vi "BEElab.vi"() -> ()   [LabVIEW 2010]
panel:
  in  "T 1":bool
  in  "T2":bool
  in  "T3":bool
  in  "T4":bool
  out "spreadsheet string":string
  in  "index 5":i32=83
  in  "index 4":i32=56
  out "error out":errorcluster
  in  "index":i32=18
  in  "index 2":i32=25
  in  "index 3":i32=52
  out "String 2":string
  out "Numeric":dbl
  out "in":i32
  out "String":string
  in  "Tab Control":enum32{"Load Profile", "View Data"}(tab)
  in  "Massachusetts - Winter":bool
  in  "Arizona  - Winter":bool
  in  "Massachusetts - Summer":bool
  in  "Arizona - Summer":bool
  out "Waveform Graph":dbl[](graph)
  in  "Weekend computer only":bool
  in  "0":dbl min=0.0 max=3.0 step=1.0
  in  "1":dbl min=0.0 max=3.0 step=1.0
  in  "2":dbl min=0.0 max=3.0 step=1.0
  in  "5":dbl min=0.0 max=3.0 step=1.0
  in  "4":dbl min=0.0 max=3.0 step=1.0
  in  "3":dbl min=0.0 max=3.0 step=1.0
  in  "11":dbl min=0.0 max=3.0 step=1.0
  in  "10":dbl min=0.0 max=3.0 step=1.0
  in  "9":dbl min=0.0 max=3.0 step=1.0
  in  "6":dbl min=0.0 max=3.0 step=1.0
  in  "7":dbl min=0.0 max=3.0 step=1.0
  in  "8":dbl min=0.0 max=3.0 step=1.0
  in  "15":dbl min=0.0 max=3.0 step=1.0
  in  "14":dbl min=0.0 max=3.0 step=1.0
  in  "13":dbl min=0.0 max=3.0 step=1.0
  in  "20":dbl min=0.0 max=3.0 step=1.0
  in  "19":dbl min=0.0 max=3.0 step=1.0
  in  "16":dbl min=0.0 max=3.0 step=1.0
  in  "17":dbl min=0.0 max=3.0 step=1.0
  in  "18":dbl min=0.0 max=3.0 step=1.0
  in  "23":dbl min=0.0 max=3.0 step=1.0
  in  "22":dbl min=0.0 max=3.0 step=1.0
  in  "21":dbl min=0.0 max=3.0 step=1.0
  in  "12":dbl min=0.0 max=3.0 step=1.0
  in  "Step Usage":bool
  in  "Office 9am - 5pm work day":bool
  in  "Launch Experiment":bool
  in  "Clear":bool
  out "Temperture":cluster{dbl, dbl, dbl, dbl}(graph)
  out "Usage Watts":cluster{dbl}(graph)
  in  "stop":bool
  out "Thermal Load Profile":dbl[](graph)
  # "Building Energy Efficiency iLab"
  # "Select the climate (currently externally controlled).\n\nUse the predefined configurations or custom configuration area\nto specify thermal load profiles for your experimnt.\n\nCLick the Save and Launch button to begin your experiment."
  # "Select a climate for the test chamber:"
  # "Predefined Configurations:"
  # "Custom Configurations:"
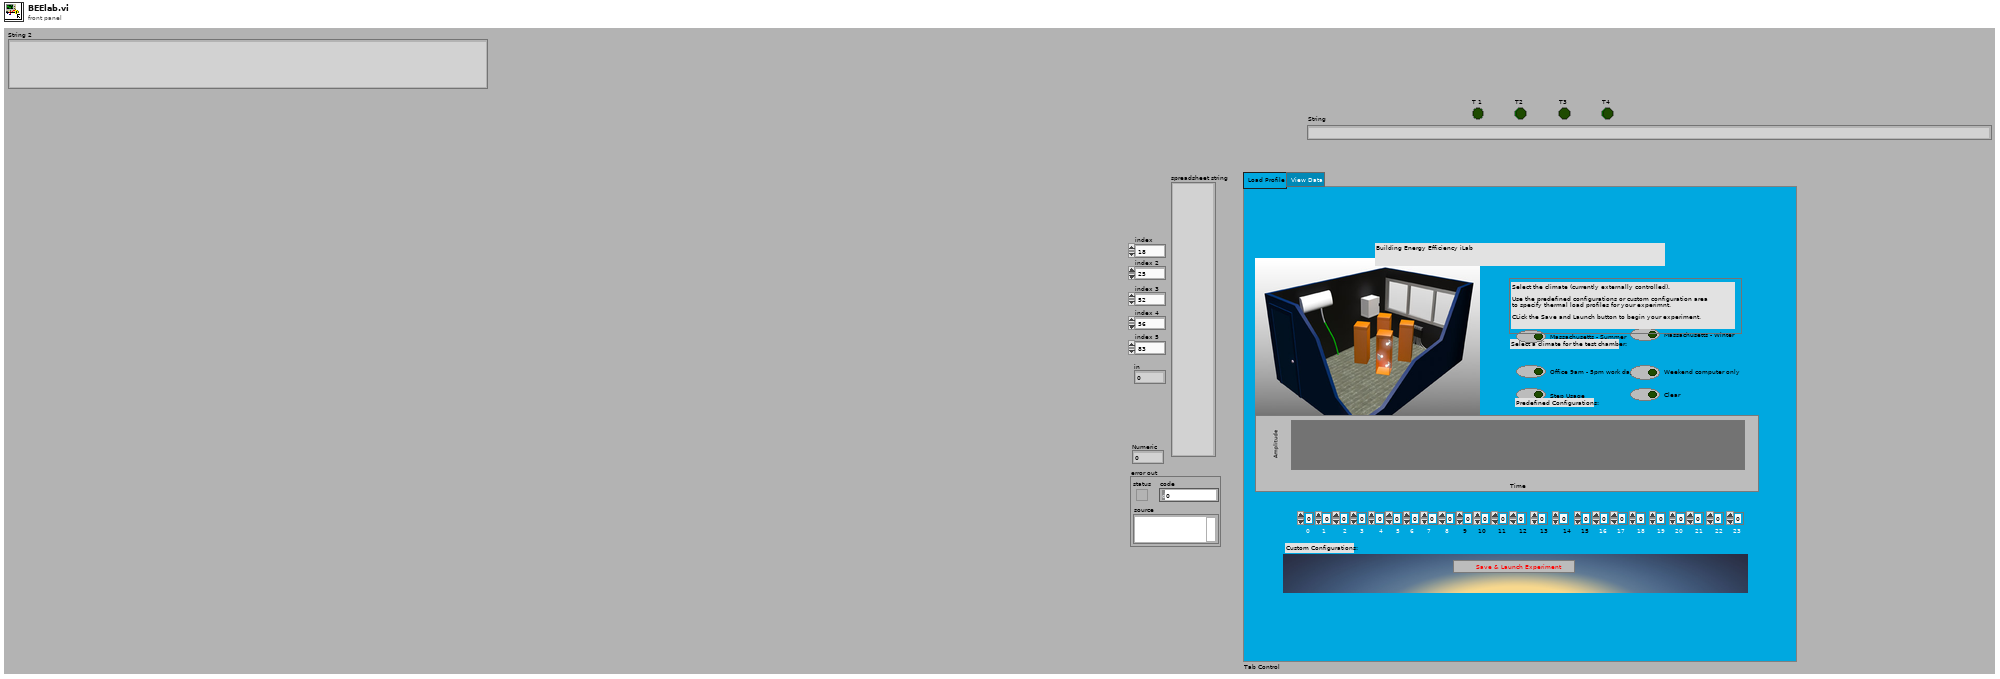
[diagram p1: front panel]
types:
  T1 = enum16{"Read", "Write", "ReadWrite", "BufferedRead", "BufferedReadWrite"}
  T2 = enum32{"Page Enabled", "Page Disabled", "Page Disabled & Grayed"}
  T3 = cluster{"0":dbl, "1":dbl, "2":dbl, "3":dbl, "4":dbl, "5":dbl, "6":dbl, "7":dbl, "8":dbl, "9":dbl, "10":dbl, "11":dbl, "12":dbl, "13":dbl, "14":dbl, "15":dbl, "16":dbl, "17":dbl, "18":dbl, "19":dbl, "20":dbl, "21":dbl, "22":dbl, "23":dbl}
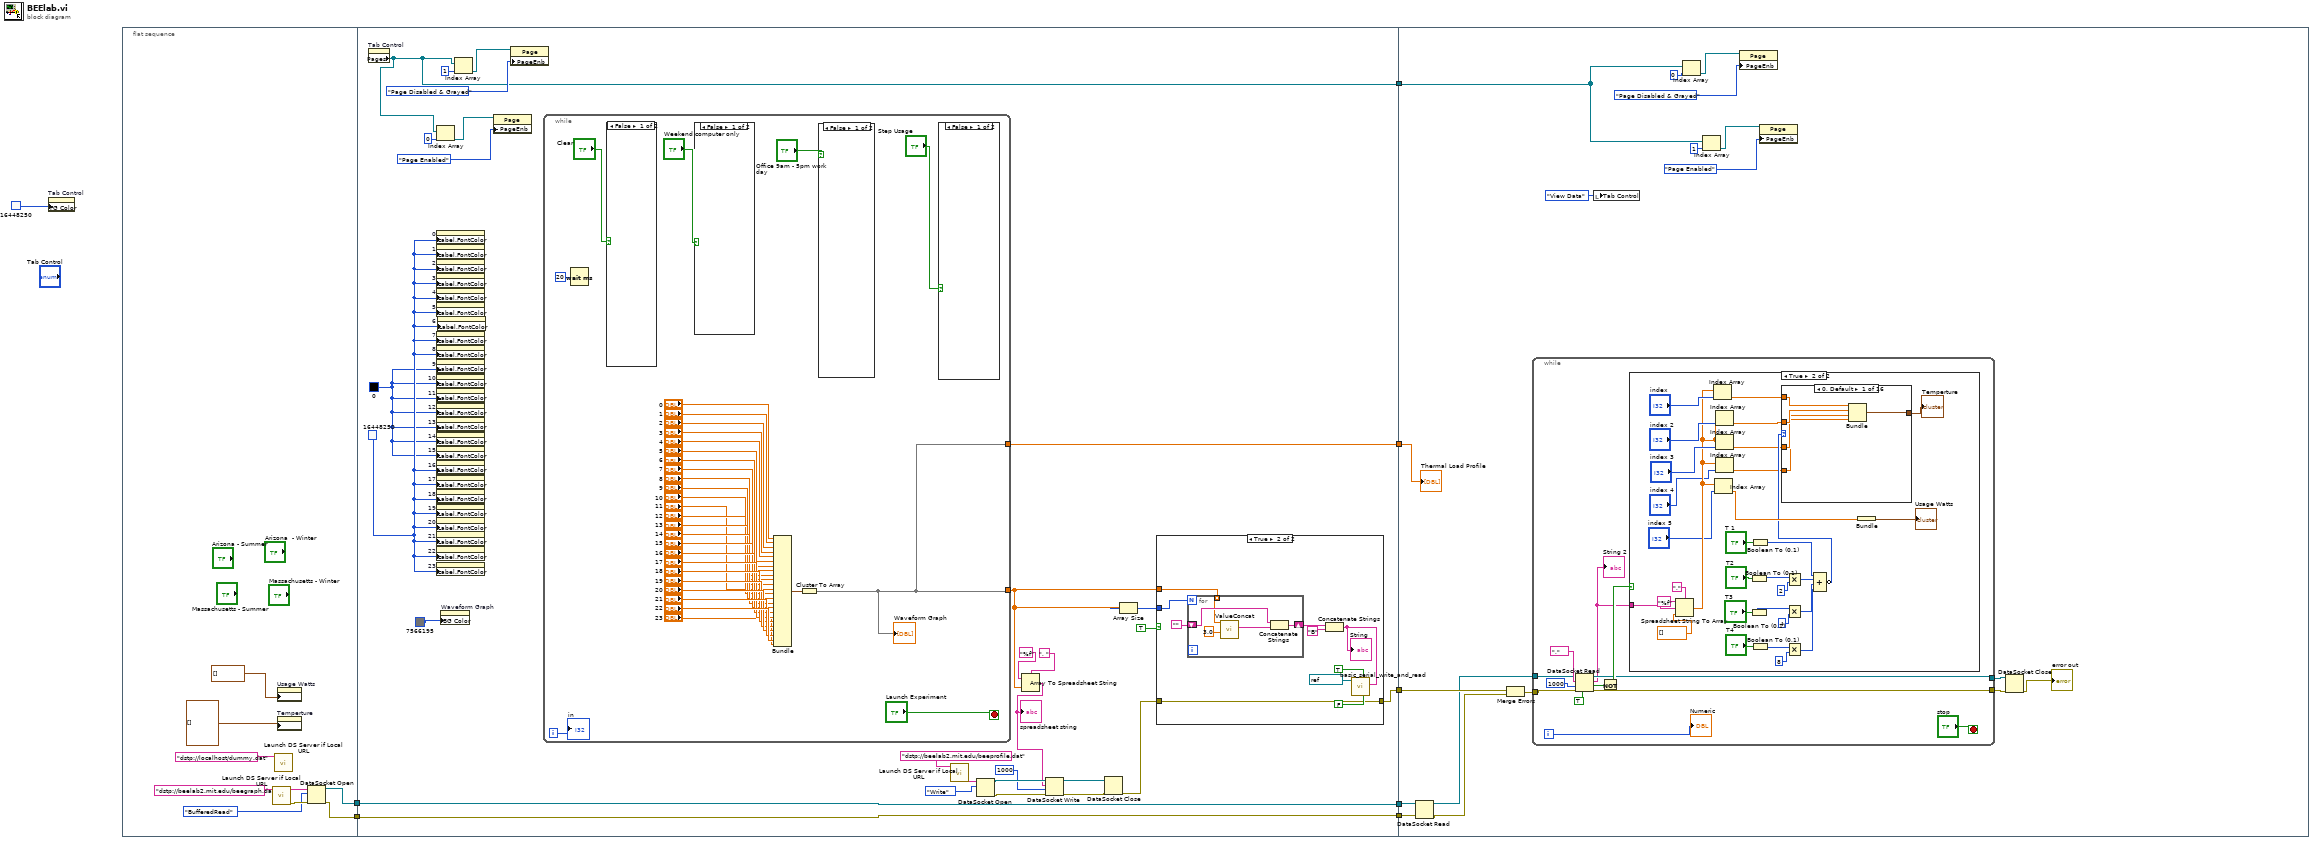
[diagram p0: block diagram]
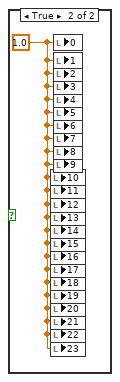
[diagram p3: hidden frame]
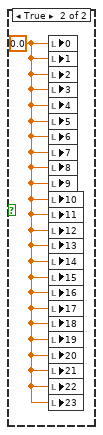
[diagram p4: hidden frame]
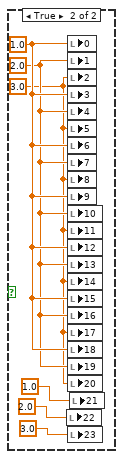
[diagram p5: hidden frame]
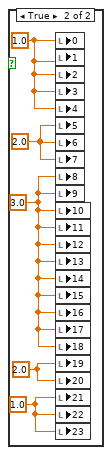
[diagram p6: hidden frame]
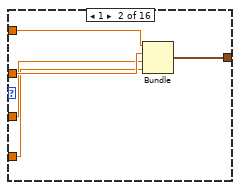
[diagram p8: hidden frame]
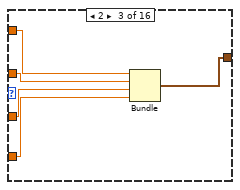
[diagram p9: hidden frame]
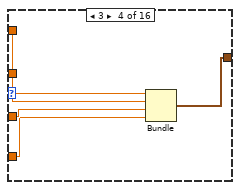
[diagram p10: hidden frame]
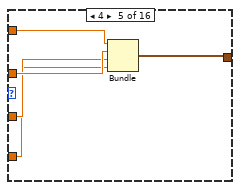
[diagram p11: hidden frame]
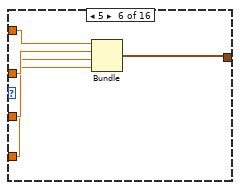
[diagram p12: hidden frame]
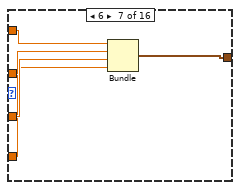
[diagram p13: hidden frame]
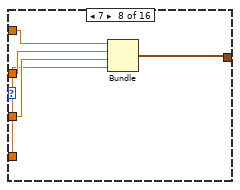
[diagram p14: hidden frame]
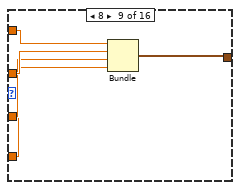
[diagram p15: hidden frame]
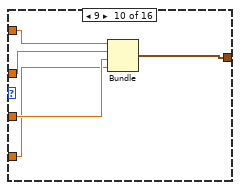
[diagram p16: hidden frame]
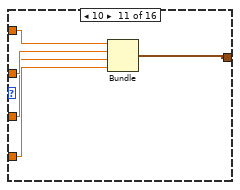
[diagram p17: hidden frame]
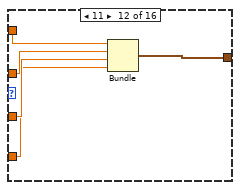
[diagram p18: hidden frame]
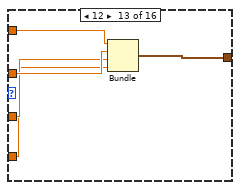
[diagram p19: hidden frame]
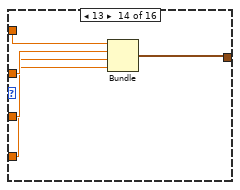
[diagram p20: hidden frame]
diagram:
  n1 = property on="Tab Control" class="TabCtl (strict)"("FG Color"=u32 16448250) -> ()  [unwired: 2 in, 2 out]
  n2 = flat-sequence {
    tunnel: [w12] -> w4
    tunnel: [w11] -> w2
    tunnel: [w36] -> w7
    tunnel: [w31] -> w6
    tunnel: [w30] -> w5
    tunnel: w4 -> [w29]
    tunnel: [w29] -> w3
    tunnel: w2 -> [w30]
    tunnel: [w18] -> w1
    tunnel: w7 -> [w122]
    tunnel: w6 -> [w115]
    tunnel: w5 -> [w110]
    tunnel: w3 -> [w109]
    tunnel: w1 -> [w114]
    frame #0 {
      n3 = call "Launch DS Server if Local URL.vi"("URL"="dstp://beelab2.mit.edu/beegraph.dat") -> ("error out"=w15:errorcluster, "Duplicate URL"=w16:string)  [unwired: 1 in, 4 out]
      n4 = call "Launch DS Server if Local URL.vi"("URL"="dstp://localhost/dummy.dat") -> ()  [unwired: 1 in, 6 out]
      n5 = property on="Usage Watts" class="WFChart (strict)"("History Data"=cluster{dbl}[] []) -> ()  [unwired: 2 in, 2 out]
      n6 = property on="Temperture" class="WFChart (strict)"("History Data"=cluster{dbl, dbl, dbl, dbl}[] []) -> ()  [unwired: 2 in, 2 out]
      n7 = DataSocket Open(8:w15, 10:T1."BufferedRead" ("mode"), 11:w16) -> (0:w12:errorcluster, 3:w11:refnum<k13>)  [unwired: 1 in]
    }
    frame #1 {
      w44 = u32 0
      w45 = u32 16448250
      n8 = property on="Tab Control" class="TabCtl (strict)"() -> ("Pages"=w36:refnum<vi>[])  [unwired: 2 in, 2 out]
      n9 = property on="15" class="DigNum (strict)"("Label.FontColor"=w44) -> ()  [unwired: 2 in, 2 out]
      n10 = property on="16" class="DigNum (strict)"("Label.FontColor"=w45) -> ()  [unwired: 2 in, 2 out]
      n11 = property on="17" class="DigNum (strict)"("Label.FontColor"=w45) -> ()  [unwired: 2 in, 2 out]
      n12 = property on="18" class="DigNum (strict)"("Label.FontColor"=w45) -> ()  [unwired: 2 in, 2 out]
      n13 = property on="19" class="DigNum (strict)"("Label.FontColor"=w45) -> ()  [unwired: 2 in, 2 out]
      n14 = property on="20" class="DigNum (strict)"("Label.FontColor"=w45) -> ()  [unwired: 2 in, 2 out]
      n15 = property on="21" class="DigNum (strict)"("Label.FontColor"=w45) -> ()  [unwired: 2 in, 2 out]
      n16 = Index Array(array=w36, index=0) -> (element=w42:refnum<vi>)
      n17 = property on="0" class="DigNum (strict)"("Label.FontColor"=w45) -> ()  [unwired: 2 in, 2 out]
      n18 = property on="1" class="DigNum (strict)"("Label.FontColor"=w45) -> ()  [unwired: 2 in, 2 out]
      n19 = property on="2" class="DigNum (strict)"("Label.FontColor"=w45) -> ()  [unwired: 2 in, 2 out]
      n20 = property on="3" class="DigNum (strict)"("Label.FontColor"=w45) -> ()  [unwired: 2 in, 2 out]
      n21 = property on="4" class="DigNum (strict)"("Label.FontColor"=w45) -> ()  [unwired: 2 in, 2 out]
      n22 = property on="5" class="DigNum (strict)"("Label.FontColor"=w45) -> ()  [unwired: 2 in, 2 out]
      n23 = property on="7" class="DigNum (strict)"("Label.FontColor"=w45) -> ()  [unwired: 2 in, 2 out]
      n24 = property on="8" class="DigNum (strict)"("Label.FontColor"=w45) -> ()  [unwired: 2 in, 2 out]
      n25 = property on="9" class="DigNum (strict)"("Label.FontColor"=w44) -> ()  [unwired: 2 in, 2 out]
      n26 = property on="10" class="DigNum (strict)"("Label.FontColor"=w44) -> ()  [unwired: 2 in, 2 out]
      n27 = property on="11" class="DigNum (strict)"("Label.FontColor"=w44) -> ()  [unwired: 2 in, 2 out]
      n28 = property on="12" class="DigNum (strict)"("Label.FontColor"=w44) -> ()  [unwired: 2 in, 2 out]
      n29 = property on="13" class="DigNum (strict)"("Label.FontColor"=w44) -> ()  [unwired: 2 in, 2 out]
      n30 = property on="14" class="DigNum (strict)"("Label.FontColor"=w44) -> ()  [unwired: 2 in, 2 out]
      n31 = property on="22" class="DigNum (strict)"("Label.FontColor"=w45) -> ()  [unwired: 2 in, 2 out]
      n32 = property on="23" class="DigNum (strict)"("Label.FontColor"=w45) -> ()  [unwired: 2 in, 2 out]
      n33 = property on="6" class="DigNum (strict)"("Label.FontColor"=w45) -> ()  [unwired: 2 in, 2 out]
      n34 = property on="Waveform Graph" class="WFGraph (strict)"("BG Color"=u32 7566195) -> ()  [unwired: 2 in, 2 out]
      n35 = Index Array(array=w36, index=1) -> (element=w41:refnum<vi>)
      n36 = property class="Page"(reference=w42, "PageEnb"=T2."Page Enabled" ("Page Enabled State")) -> ()  [unwired: 1 in, 2 out]
      n37 = property class="Page"(reference=w41, "PageEnb"=T2."Page Disabled & Grayed" ("Page Enabled State")) -> ()  [unwired: 1 in, 2 out]
      n38 = while {
        tunnel: [w63] -> w35
        tunnel: [w63] -> w18
        i -> [w66]
        stop <- "Launch Experiment" stop-if-true
        n39 = Wait (ms)(milliseconds to wait=u32 20) -> ()  [unwired: 1 out]
        n40 = case shown="False" "Clear" {
          frame False {
          }
          frame True {
            w97 = 0.0 ("0")
            n41 = local write "0"(w97) -> ()
            n42 = local write "1"(w97) -> ()
            n43 = local write "2"(w97) -> ()
            n44 = local write "3"(w97) -> ()
            n45 = local write "4"(w97) -> ()
            n46 = local write "5"(w97) -> ()
            n47 = local write "6"(w97) -> ()
            n48 = local write "7"(w97) -> ()
            n49 = local write "8"(w97) -> ()
            n50 = local write "9"(w97) -> ()
            n51 = local write "10"(w97) -> ()
            n52 = local write "11"(w97) -> ()
            n53 = local write "12"(w97) -> ()
            n54 = local write "13"(w97) -> ()
            n55 = local write "14"(w97) -> ()
            n56 = local write "15"(w97) -> ()
            n57 = local write "16"(w97) -> ()
            n58 = local write "17"(w97) -> ()
            n59 = local write "18"(w97) -> ()
            n60 = local write "19"(w97) -> ()
            n61 = local write "20"(w97) -> ()
            n62 = local write "21"(w97) -> ()
            n63 = local write "22"(w97) -> ()
            n64 = local write "23"(w97) -> ()
          }
        }
        n65 = case shown="False" "Weekend computer only" {
          frame False {
          }
          frame True {
            w96 = 1.0 ("0")
            n66 = local write "10"(w96) -> ()
            n67 = local write "11"(w96) -> ()
            n68 = local write "12"(w96) -> ()
            n69 = local write "13"(w96) -> ()
            n70 = local write "14"(w96) -> ()
            n71 = local write "15"(w96) -> ()
            n72 = local write "16"(w96) -> ()
            n73 = local write "17"(w96) -> ()
            n74 = local write "18"(w96) -> ()
            n75 = local write "19"(w96) -> ()
            n76 = local write "20"(w96) -> ()
            n77 = local write "21"(w96) -> ()
            n78 = local write "22"(w96) -> ()
            n79 = local write "23"(w96) -> ()
            n80 = local write "0"(w96) -> ()
            n81 = local write "1"(w96) -> ()
            n82 = local write "2"(w96) -> ()
            n83 = local write "3"(w96) -> ()
            n84 = local write "4"(w96) -> ()
            n85 = local write "5"(w96) -> ()
            n86 = local write "6"(w96) -> ()
            n87 = local write "7"(w96) -> ()
            n88 = local write "8"(w96) -> ()
            n89 = local write "9"(w96) -> ()
          }
        }
        n90 = Bundle("0"="0", "1"="1", "2"="2", "3"="3", "4"="4", "5"="5", "6"="6", "7"="7", "8"="8", "9"="9", "10"="10", "11"="11", "12"="12", "13"="13", "14"="14", "15"="15", "16"="16", "17"="17", "18"="18", "19"="19", "20"="20", "21"="21", "22"="22", "23"="23") -> (w72:T3)  [unwired: 1 in]
        n91 = Cluster To Array(cluster=w72) -> (array=w63:dbl[])
        "Waveform Graph" <- w63
        n92 = case shown="False" "Office 9am - 5pm work day" {
          frame False {
          }
          frame True {
            w104 = 1.0 ("21")
            w105 = 2.0 ("19")
            w106 = 3.0 ("8")
            w107 = 2.0 ("5")
            w108 = 1.0 ("0")
            n93 = local write "0"(w108) -> ()
            n94 = local write "1"(w108) -> ()
            n95 = local write "2"(w108) -> ()
            n96 = local write "3"(w108) -> ()
            n97 = local write "4"(w108) -> ()
            n98 = local write "5"(w107) -> ()
            n99 = local write "6"(w107) -> ()
            n100 = local write "7"(w107) -> ()
            n101 = local write "8"(w106) -> ()
            n102 = local write "9"(w106) -> ()
            n103 = local write "10"(w106) -> ()
            n104 = local write "11"(w106) -> ()
            n105 = local write "12"(w106) -> ()
            n106 = local write "13"(w106) -> ()
            n107 = local write "14"(w106) -> ()
            n108 = local write "15"(w106) -> ()
            n109 = local write "16"(w106) -> ()
            n110 = local write "17"(w106) -> ()
            n111 = local write "18"(w106) -> ()
            n112 = local write "19"(w105) -> ()
            n113 = local write "20"(w105) -> ()
            n114 = local write "21"(w104) -> ()
            n115 = local write "22"(w104) -> ()
            n116 = local write "23"(w104) -> ()
          }
        }
        n117 = case shown="False" "Step Usage" {
          frame False {
          }
          frame True {
            w101 = 3.0 ("2")
            w102 = 2.0 ("1")
            w103 = 1.0 ("0")
            n118 = local write "22"(2.0 ("22")) -> ()
            n119 = local write "0"(w103) -> ()
            n120 = local write "1"(w102) -> ()
            n121 = local write "2"(w101) -> ()
            n122 = local write "3"(w103) -> ()
            n123 = local write "4"(w102) -> ()
            n124 = local write "5"(w101) -> ()
            n125 = local write "6"(w103) -> ()
            n126 = local write "7"(w102) -> ()
            n127 = local write "8"(w101) -> ()
            n128 = local write "9"(w103) -> ()
            n129 = local write "10"(w102) -> ()
            n130 = local write "11"(w101) -> ()
            n131 = local write "12"(w103) -> ()
            n132 = local write "13"(w102) -> ()
            n133 = local write "14"(w101) -> ()
            n134 = local write "15"(w103) -> ()
            n135 = local write "16"(w102) -> ()
            n136 = local write "17"(w101) -> ()
            n137 = local write "18"(w103) -> ()
            n138 = local write "19"(w102) -> ()
            n139 = local write "20"(w101) -> ()
            n140 = local write "23"(3.0 ("22")) -> ()
            n141 = local write "21"(1.0 ("21")) -> ()
          }
        }
        "in" <- w66
      }
      n142 = call "Launch DS Server if Local URL.vi"("URL"="dstp://beelab2.mit.edu/beeprofile.dat") -> ("Duplicate URL"=w25:string)  [unwired: 1 in, 5 out]
      n143 = DataSocket Open(10:T1."Write" ("mode"), 11:w25) -> (0:w22:errorcluster, 3:w23:refnum<k13>)  [unwired: 2 in]
      n144 = Array To Spreadsheet String(delimiter (Tab)=", ", array=w35, 3:"%f" ("format string")) -> (spreadsheet string=w19:string)
      "spreadsheet string" <- w19
      n145 = DataSocket Write(8:w22, 9:1000 ("ms timeout (0)"), 10:w19, 11:w23) -> (0:w27:errorcluster, 3:w28:refnum<k13>)  [unwired: 1 out]
      n146 = DataSocket Close(8:w27, 11:w28) -> (0:w21:errorcluster)  [unwired: 1 in, 1 out]
      n147 = Array Size(array=w35) -> (size(s)=w46:i32)
      n148 = case shown="True" TRUE {
        tunnel: w46 -> [_ w50]
        tunnel: w35 -> [_ w49]
        tunnel: w21 -> [w47 w48]
        tunnel: [w47 w48] -> w31
        frame False {
        }
        frame True {
          n149 = for {
            N: w50 -> [_]
            shift-right: [w62] -> w56
            shift-left: "" -> [w61]
            tunnel: w49 -> [w58] mode=indexing
            n150 = call "ValueConcat.vi"("Length"=3.0, "Value"=w58) -> ("Output"=w60:string)  [unwired: 9 in]
            n151 = Concatenate Strings(w61, w60) -> (w62:string)
          }
          n152 = Concatenate Strings(w56, "B" ("string")) -> (w57:string)
          "String" <- w57
          n153 = call "basic_serial_write_and_read.vi"("VISA resource name"=refnum<visa-resource-name> "COM7", "write"=TRUE, "read"=FALSE, "string to write"=w57) -> ()  [unwired: 6 in, 1 out]
        }
      }
    }
    frame #2 {
      n154 = DataSocket Read(8:w109, 11:w110) -> (0:w111:errorcluster, 3:w112:refnum<k13>)  [unwired: 3 in, 5 out]
      n155 = Merge Errors(w115, w111) -> (w116:errorcluster)
      n156 = while {
        tunnel: [w133] -> w118
        tunnel: [w132] -> w119
        tunnel: w116 -> [w127]
        tunnel: w112 -> [w128]
        i -> [w129]
        stop <- "stop" stop-if-true
        n157 = DataSocket Read(6:TRUE ("wait for updated value (T)"), 8:w127, 9:1000 ("ms timeout (10000)"), 10:",", 11:w128) -> (0:w132:errorcluster, 1:w136:bool, 2:w131:string, 3:w133:refnum<k13>)  [unwired: 3 out]
        "String 2" <- w131
        n158 = Not(x=w136) -> (.not. x?=w135:bool)
        n159 = case shown="True" w135 {
          tunnel: w131 -> [_ w170]
          frame False {
          }
          frame True {
            n160 = Spreadsheet String To Array(delimiter (Tab)=",", format string="%f", spreadsheet string=w170, array type (2D Dbl)=dbl[] []) -> (array=w163:dbl[])
            n161 = Index Array(array=w163, index="index") -> (element=w144:dbl)
            n162 = Index Array(array=w163, index="index 5") -> (element=w157:dbl)
            n163 = Index Array(array=w163, index="index 2") -> (element=w143:dbl)
            n164 = Index Array(array=w163, index="index 3") -> (element=w142:dbl)
            n165 = Index Array(array=w163, index="index 4") -> (element=w141:dbl)
            n166 = Boolean To (0,1)(Boolean="T2") -> (0, 1=w152:i16)
            n167 = Boolean To (0,1)(Boolean="T3") -> (0, 1=w151:i16)
            n168 = Boolean To (0,1)(Boolean="T 1") -> (0, 1=w146:i16)
            n169 = Boolean To (0,1)(Boolean="T4") -> (0, 1=w150:i16)
            n170 = Multiply(x=w152, y=2) -> (x*y=w147:i32)
            n171 = Multiply(x=w151, y=4) -> (x*y=w148:i32)
            n172 = Multiply(x=w150, y=8) -> (x*y=w149:i32)
            n173 = Compound Arithmetic op=ADD(w146, w147, w148, w149) -> (invert w145:i32)
            n174 = case shown="0, Default" w145 {
              tunnel: w144 -> [w175 w180 w185 w190 w195 w200 w205 w210 w215 w220 w225 w230 w235 w240 w245 w250]
              tunnel: w143 -> [w174 w179 w184 w189 w194 w199 w204 w209 w214 w219 w224 w229 w234 w239 w244 w249]
              tunnel: w142 -> [w173 w178 w183 w188 w193 w198 w203 w208 w213 w218 w223 w228 w233 w238 w243 w248]
              tunnel: w141 -> [w172 w177 w182 w187 w192 w197 w202 w207 w212 w217 w222 w227 w232 w237 w242 w247]
              tunnel: [w171 w176 w181 w186 w191 w196 w201 w206 w211 w216 w221 w226 w231 w236 w241 w246] -> w140
              frame 0, Default {
                n175 = Bundle(w175, w174, w173, w172) -> (w171:cluster{dbl, dbl, dbl, dbl})  [unwired: 1 in]
              }
              frame 1 {
                n176 = Bundle(w180, w179, w178, w177) -> (w176:cluster{dbl, dbl, dbl, dbl})  [unwired: 1 in]
              }
              frame 2 {
                n177 = Bundle(w185, w184, w183, w182) -> (w181:cluster{dbl, dbl, dbl, dbl})  [unwired: 1 in]
              }
              frame 3 {
                n178 = Bundle(w190, w189, w188, w187) -> (w186:cluster{dbl, dbl, dbl, dbl})  [unwired: 1 in]
              }
              frame 4 {
                n179 = Bundle(w195, w194, w193, w192) -> (w191:cluster{dbl, dbl, dbl, dbl})  [unwired: 1 in]
              }
              frame 5 {
                n180 = Bundle(w200, w199, w198, w197) -> (w196:cluster{dbl, dbl, dbl, dbl})  [unwired: 1 in]
              }
              frame 6 {
                n181 = Bundle(w205, w204, w203, w202) -> (w201:cluster{dbl, dbl, dbl, dbl})  [unwired: 1 in]
              }
              frame 7 {
                n182 = Bundle(w210, w209, w208, w207) -> (w206:cluster{dbl, dbl, dbl, dbl})  [unwired: 1 in]
              }
              frame 8 {
                n183 = Bundle(w215, w214, w213, w212) -> (w211:cluster{dbl, dbl, dbl, dbl})  [unwired: 1 in]
              }
              frame 9 {
                n184 = Bundle(w220, w219, w218, w217) -> (w216:cluster{dbl, dbl, dbl, dbl})  [unwired: 1 in]
              }
              frame 10 {
                n185 = Bundle(w225, w224, w223, w222) -> (w221:cluster{dbl, dbl, dbl, dbl})  [unwired: 1 in]
              }
              frame 11 {
                n186 = Bundle(w230, w229, w228, w227) -> (w226:cluster{dbl, dbl, dbl, dbl})  [unwired: 1 in]
              }
              frame 12 {
                n187 = Bundle(w235, w234, w233, w232) -> (w231:cluster{dbl, dbl, dbl, dbl})  [unwired: 1 in]
              }
              frame 13 {
                n188 = Bundle(w240, w239, w238, w237) -> (w236:cluster{dbl, dbl, dbl, dbl})  [unwired: 1 in]
              }
              frame 14 {
                n189 = Bundle(w245, w244, w243, w242) -> (w241:cluster{dbl, dbl, dbl, dbl})  [unwired: 1 in]
              }
              frame 15 {
                n190 = Bundle(w250, w249, w248, w247) -> (w246:cluster{dbl, dbl, dbl, dbl})  [unwired: 1 in]
              }
            }
            "Temperture" <- w140
            n191 = Bundle(w157) -> (→"Usage Watts":cluster{dbl})  [unwired: 1 in]
          }
        }
        "Numeric" <- w129
      }
      n192 = local write "Tab Control"(enum32{"Load Profile", "View Data"}."View Data" ("Tab Control")) -> ()
      n193 = Index Array(array=w122, index=0) -> (element=w120:refnum<vi>)
      n194 = Index Array(array=w122, index=1) -> (element=w121:refnum<vi>)
      n195 = property class="Page"(reference=w120, "PageEnb"=T2."Page Disabled & Grayed" ("Page Enabled State")) -> ()  [unwired: 1 in, 2 out]
      n196 = property class="Page"(reference=w121, "PageEnb"=T2."Page Enabled" ("Page Enabled State")) -> ()  [unwired: 1 in, 2 out]
      n197 = DataSocket Close(8:w119, 11:w118) -> (0:→"error out":errorcluster)  [unwired: 1 in, 1 out]
      "Thermal Load Profile" <- w114
    }
  }
